vi "Bool Array to Num.vi"(9 "New Bool Array":bool[](array[boolean]), 11 "Old Bool Array":bool[](array[boolean])) -> (3 "Value":u8)   [LabVIEW 2017, in "2D Plot.lvclass"]
uses:
  <vilib>/Math Plots/2D Math Plots/2D Plot/2D Plot/2D Plot.lvclass
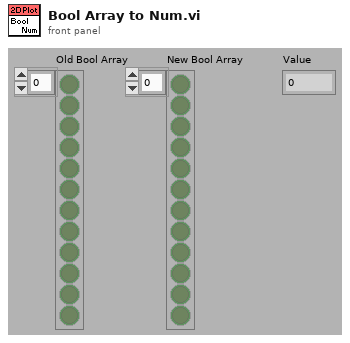
[diagram p1: front panel]
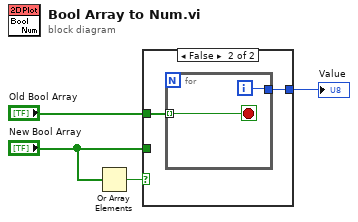
[diagram p0: block diagram]
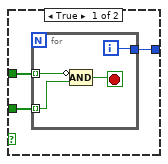
[diagram p2: hidden frame]
diagram:
  n1 = Or Array Elements(Boolean array="New Bool Array") -> (logical OR=w2:bool)
  n2 = case shown="False" w2 {
    tunnel: [w7 w13] -> w4
    tunnel: "Old Bool Array" -> [w6 w12]
    tunnel: "New Bool Array" -> [w5 _]
    frame True {
      n3 = for {
        tunnel: w6 -> [w11] mode=indexing
        tunnel: w5 -> [w10] mode=indexing
        tunnel: [w8] -> w7
        i -> [w8]
        stop <- w9 stop-if-true
        n4 = Compound Arithmetic op=AND(invert w11, w10) -> (w9:bool)
      }
    }
    frame False {
      n5 = for {
        tunnel: w12 -> [w14] mode=indexing
        tunnel: [w15] -> w13
        i -> [w15]
        stop <- w14 stop-if-true
      }
    }
  }
  "Value" <- w4
